vi "New Rotating Daily File Sink.vi"(8 "error in (no error)":errorcluster, 10 "Time to Rotate":timestamp format="%<%H:%M>T", 11 "File Path":path) -> (0 "error out":errorcluster, 3 "Rotating Daily File Sink out":refnum<class "Rotating Daily File Sink.lvclass">)   [LabVIEW 2020, in "LV Log.lvlib" / "Rotating Daily File Sink.lvclass"]
uses:
  Rotating Daily File Sink.lvclass
  Rotating Daily File Sink.lvclass/Rotating Daily File Sink.ctl
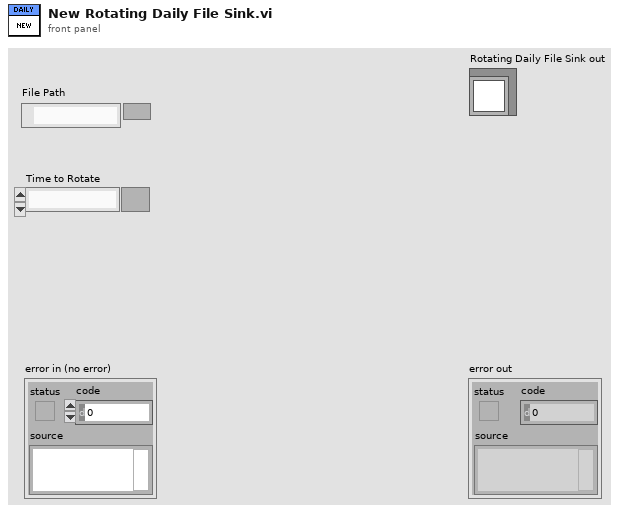
[diagram p1: front panel]
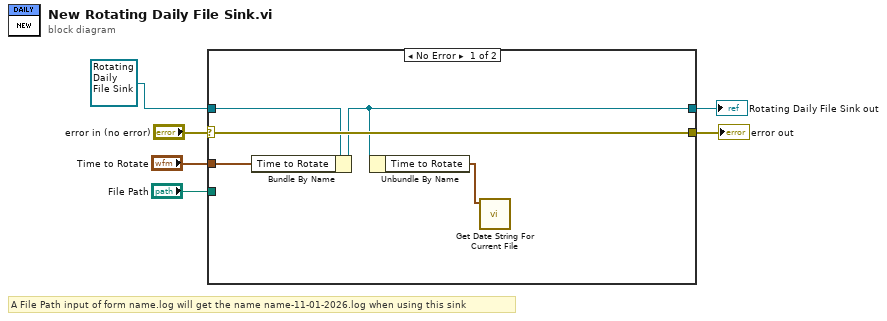
[diagram p0: block diagram]
diagram:
  # "A File Path input of form name.log will get the name name-11-01-2026.log when using this sink"
  n1 = case shown="No Error" "error in (no error)" {
    selector: "error in (no error)" -> [w11 w13]
    tunnel: [w11 w13] -> w6
    tunnel: [w8 w12] -> w4
    tunnel: refnum<class "Rotating Daily File Sink.lvclass"> refnum ("Rotating Daily File Sink out") -> [w10 w12]
    tunnel: "Time to Rotate" -> [w9 _]
    tunnel: "File Path" -> [_ _]
    frame No Error {
      n2 = Bundle By Name(cluster=w10, "Time to Rotate"=w9) -> (w8:refnum<class "Rotating Daily File Sink.lvclass">)
      n3 = Unbundle By Name(w8) -> ("Time to Rotate"=w7:timestamp)
      n4 = call "Get Date String For Current File.vi"("Time to Rotate"=w7) -> ()  [unwired: 11 in]
    }
    frame Error {
    }
  }
  "error out" <- w6
  "Rotating Daily File Sink out" <- w4
